vi "CreateResultTree.vi"(8 "error in (no error)":errorcluster, 10 "Tree Refnum":refnum<vi>) -> (0 "error out":errorcluster, 3 "ResultTree out":refnum<class "ResultTree.lvclass">)   [LabVIEW 2019, in "ResultTree.lvclass"]
doc: "Creates a new <B>ResultTree</B>. Clears all items currently in the tree and sets the default column headers."
uses:
  ResultTree.lvclass
  ResultTree.lvclass/ResultTree.ctl
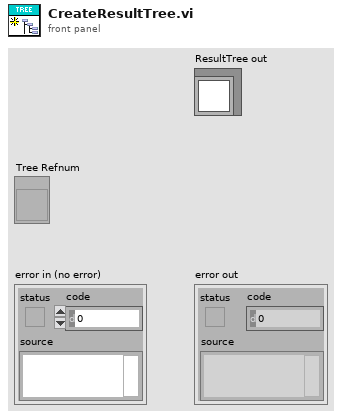
[diagram p1: front panel]
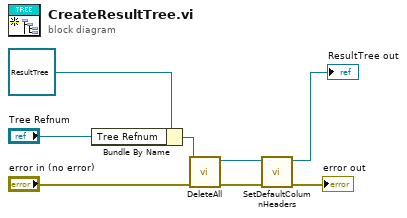
[diagram p0: block diagram]
diagram:
  n1 = Bundle By Name(cluster=refnum<class "ResultTree.lvclass"> refnum ("ResultTree in"), "Tree Refnum"="Tree Refnum") -> (w4:refnum<class "ResultTree.lvclass">)
  n2 = call "DeleteAll.vi"("error in (no error)"="error in (no error)", "ResultTree in"=w4) -> ("error out"=w7:errorcluster, "ResultTree out"=w2:refnum<class "ResultTree.lvclass">)  [unwired: 8 in]
  n3 = call "SetDefaultColumnHeaders.vi"("error in (no error)"=w7, "ResultTree in"=w2) -> ("error out"=→"error out":errorcluster, "ResultTree out"=→"ResultTree out":refnum<class "ResultTree.lvclass">)  [unwired: 8 in]
